vi "setUp.vi"(8 "error in (no error)":errorcluster, 11 "reference in":refnum<class "GUI Interlock Tester.lvclass">) -> (0 "error out":errorcluster, 3 "reference out":refnum<class "GUI Interlock Tester.lvclass">)   [LabVIEW 2018, in "GUI Interlock Tester.lvclass"]
doc: "setUp runs prior to the test method during test execution. Use this method to initialize any object data required by your tests."
uses:
  GUI Interlock Tester.lvclass
  C:/Program Files (x86)/National Instruments/LabVIEW 2018/vi.lib/addons/_JKI Toolkits/VI Tester/TestCase.llb/TestCase.lvclass
  GUI Interlock Tester.lvclass/GUI Interlock Tester.ctl
  <vilib>/addons/_JKI Toolkits/VI Tester/TestCase.llb/TestCase.lvclass
panel:
  in  "Self Test Button":bool
  in  "Power Off Button":bool
  in  "Power On Button":bool
  # "The buttons below are not intended to be inputs. Their role is to be \npassed by this VI via the output \"reference out\"."
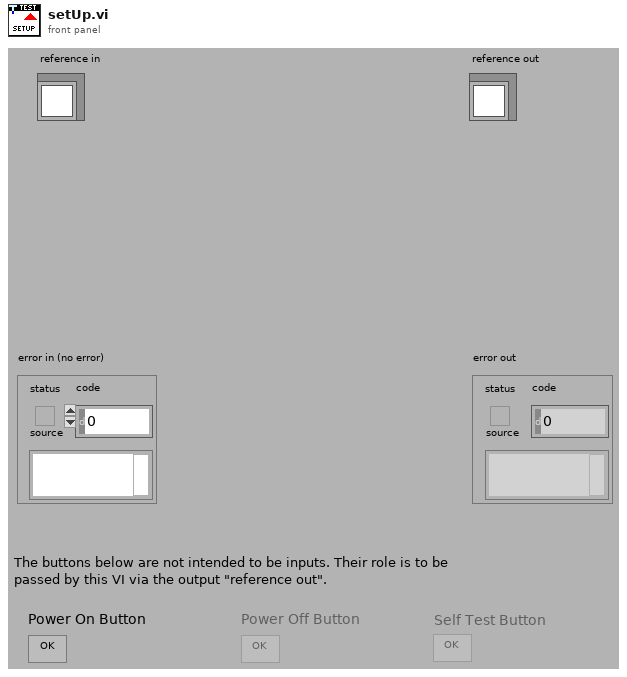
[diagram p1: front panel]
types:
  T1 = enum8{"Enabled", "Disabled", "Disabled and Grayed Out"}
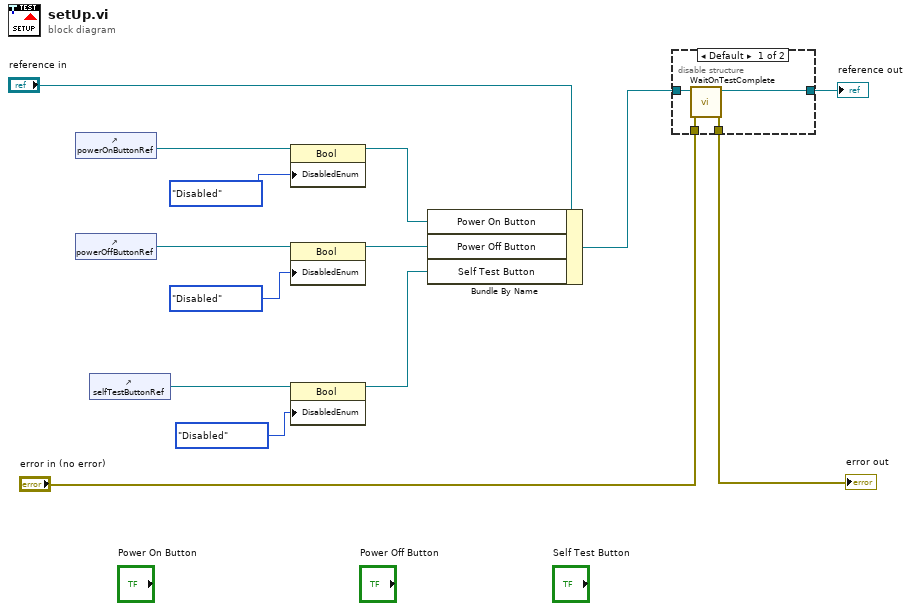
[diagram p0: block diagram]
diagram:
  n1 = control-ref of="powerOnButtonRef"() -> (w9:refnum<vi>)
  n2 = control-ref of="powerOffButtonRef"() -> (w6:refnum<vi>)
  n3 = control-ref of="selfTestButtonRef"() -> (w5:refnum<vi>)
  n4 = property class="Bool"(reference=w9, "DisabledEnum"=T1."Disabled" ("Disabled")) -> (reference out=w3:refnum<vi>)  [unwired: 1 in, 1 out]
  n5 = property class="Bool"(reference=w6, "DisabledEnum"=T1."Disabled" ("Disabled")) -> (reference out=w2:refnum<vi>)  [unwired: 1 in, 1 out]
  n6 = property class="Bool"(reference=w5, "DisabledEnum"=T1."Disabled" ("Disabled")) -> (reference out=w1:refnum<vi>)  [unwired: 1 in, 1 out]
  n7 = Bundle By Name(cluster="reference in", "Power On Button"=w3, "Power Off Button"=w2, "Self Test Button"=w1) -> (w10:refnum<class "GUI Interlock Tester.lvclass">)
  n8 = disable-structure shown="Default" {
    disable-tunnel: "error in (no error)" -> [w18 w19]
    disable-tunnel: [w17 w19] -> w13
    disable-tunnel: [w16 w20] -> w11
    disable-tunnel: w10 -> [w15 w20]
    frame condition #0 (active) {
      n9 = call <vilib>:"WaitOnTestComplete.vi"("error in (no error)"=w18, "TestCase in"=w15) -> ("error out"=w17:errorcluster, "TestCase out"=w16:refnum<class "GUI Interlock Tester.lvclass">)  [unwired: 8 in]
    }
    frame condition #1 {
    }
  }
  "error out" <- w13
  "reference out" <- w11
